vi "WPI_SolenoidSetEnum.vi"(8 "error in (no error)":errorcluster, 10 "Value":T1, 11 "SolenoidDevRef":T2={"DevStatus"={"status"=FALSE, "code"=0, "source"=""}, "Pneumatics Control Module"=0, "Forward Solenoid Channel"=enum."Invalid", "Reverse Solenoid Channel"=enum."Invalid"}) -> (0 "error out":errorcluster, 3 "SolenoidDevRef":T2={"DevStatus"={"status"=FALSE, "code"=0, "source"=""}, "Pneumatics Control Module"=0, "Forward Solenoid Channel"=enum."Invalid", "Reverse Solenoid Channel"=enum."Invalid"})   [LabVIEW 2017]
doc: "Sets the solenoid to Off, On, Forward, or Reverse. You also can wire a boolean data type to the <B>Value</B> input so that this VI specifies, when TRUE, to turn on a Single solenoid.\n\nThis software is licensed. Open the labview\\readme\\WPI Robotics Library Open Source License.txt file for more information."
uses:
  <vilib>/Rock Robotics/WPI/Solenoid/WPI_SolenoidDevRef.ctl
  <vilib>/Rock Robotics/WPI/Solenoid/WPI_SolenoidChannel.ctl
  <vilib>/Rock Robotics/WPI/Solenoid/WPI_SolenoidValue.ctl
  <vilib>/Rock Robotics/WPI/Solenoid/WPI_SolenoidCacheOp.ctl
  <vilib>/Rock Robotics/WPI/CAN/PCM/WPI_CAN_PCMGlobalOps.ctl
  <vilib>/Rock Robotics/WPI/Solenoid/WPI_SolenoidSafetyCheck.vi
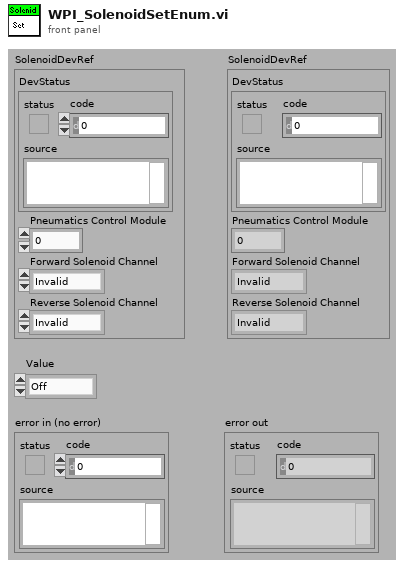
[diagram p1: front panel]
types:
  T1 = typedef "WPI_SolenoidValue.ctl" = enum16{"Off", "On", "Forward", "Reverse"}
  T2 = typedef "WPI_SolenoidDevRef.ctl" = cluster{"DevStatus":errorcluster, "Pneumatics Control Module":u8, "Forward Solenoid Channel":T3, "Reverse Solenoid Channel":T3}
  T3 = typedef "WPI_SolenoidChannel.ctl" = enum8{"Solenoid 0", "Solenoid 1", "Solenoid 2", "Solenoid 3", "Solenoid 4", "Solenoid 5", "Solenoid 6", "Solenoid 7", "Invalid"}
  T4 = typedef "WPI_SolenoidCacheOp.ctl" = enum16{"Acquire", "Release", "Status"}
  T5 = typedef "WPI_CAN_PCMGlobalOps.ctl" = enum16{"Read For Send", "Write After Receive", "Set Solenoids", "Set Closed Loop", "Clear Sticky Faults", "Get All", "Write Error", "Write After Receive Blacklist", "Set Control Frame Rate"}
  T6 = cluster{"Solenoid Status":bool[], "Battery Voltage":dbl, "Solenoid Voltage":dbl, "Compressor Current":dbl, "CompressorEnabled":bool, "StickySolenoidFault":bool, "StickyCompressorFault":bool, "SolenoidFault":bool, "CompressorFault":bool, "HardwareFault":bool, "ClosedLoopStatus":bool, "PressureStatus":bool, "Module Enabled":bool, "ClosedLoopSuggestedOutput":bool, "CAN Error":errorcluster, "Sticky Solenoid Faults":bool[]}
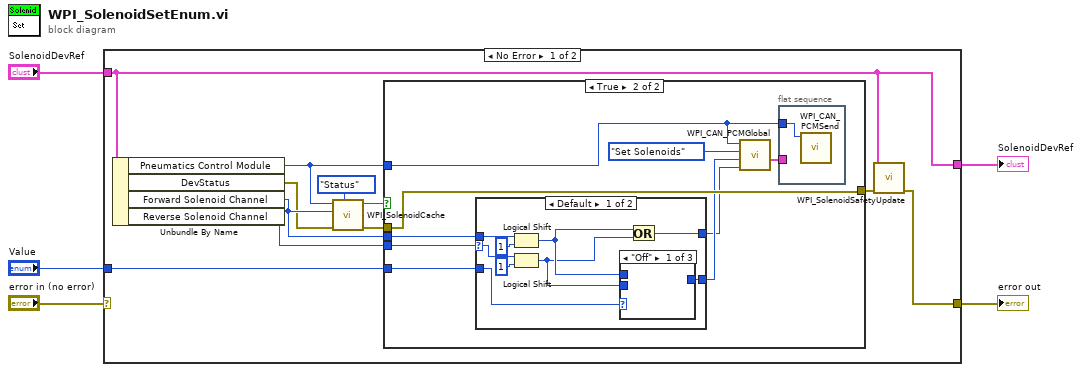
[diagram p0: block diagram]
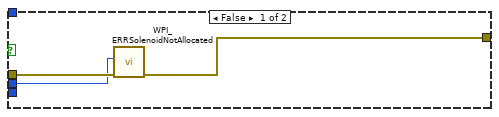
[diagram p2: hidden frame]
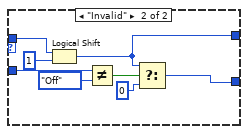
[diagram p5: hidden frame]
diagram:
  n1 = case shown="No Error" "error in (no error)" {
    selector: "error in (no error)" -> [_ w50]
    tunnel: "SolenoidDevRef" -> [w6 w49]
    tunnel: "Value" -> [w16 _]
    tunnel: [w8 w50] -> w2
    tunnel: [w6 w49] -> w1
    frame No Error {
      n2 = Unbundle By Name(w6) -> ("Pneumatics Control Module"=w15:u8, "DevStatus"=w13:errorcluster, "Forward Solenoid Channel"=w14:T3, "Reverse Solenoid Channel"=w7:T3)
      n3 = call <vilib>:"WPI_SolenoidCache.vi"("AllocatedSolenoidOp"=WPI_SolenoidCacheOp."Status", "error in (no error)"=w13, "SolenoidChannel"=w14, "Pneumatics Control Module"=w15) -> ("error out"=w11:errorcluster, "Allocated"=w12:bool)  [unwired: 6 out]
      n4 = case shown="True" w12 {
        tunnel: w16 -> [_ w28]
        tunnel: [w19 w24] -> w9
        tunnel: w15 -> [_ w21]
        tunnel: w14 -> [w17 w27]
        tunnel: w11 -> [w18 w24]
        tunnel: w7 -> [_ w26]
        frame False {
          n5 = call <vilib>:"WPI_ERRSolenoidNotAllocated.vi"("error in (no error)"=w18, "Solenoid Channel"=w17) -> ("error out"=w19:errorcluster)  [unwired: 9 in]
        }
        frame True {
          n6 = case shown="Default" w26 {
            selector: w26 -> [w35 _]
            tunnel: w28 -> [w34 w46]
            tunnel: [w33 w42] -> w23
            tunnel: w27 -> [w37 w47]
            tunnel: [w30 w43] -> w22
            frame Default {
              n7 = Logical Shift(y=w37, x=u8 1) -> (x << y=w32:u8)
              n8 = Logical Shift(y=w35, x=u8 1) -> (x << y=w31:u8)
              n9 = case shown="\"Off\"" w34 {
                tunnel: w32 -> [_ w39 _]
                tunnel: w31 -> [_ _ w40]
                tunnel: [_ w39 w40] -> w33
                frame "Off" {
                }
                frame "Forward", Default {
                }
                frame "Reverse" {
                }
              }
              n10 = Or(x=w32, y=w31) -> (x .or. y?=w30:u8)
            }
            frame "Invalid" {
              n11 = Logical Shift(y=w47, x=u8 1) -> (x << y=w43:u8)
              n12 = Not Equal?(x=w46, y=WPI_SolenoidValue."Off") -> (x != y?=w44:bool)
              n13 = Select(t=w43, s=w44, f=u8 0) -> (s? t:f=w42:u8)
            }
          }
          n14 = call <vilib>:"WPI_CAN_PCMGlobal.vi"("Solenoid Set Mask"=w22, "Solenoid Set Value"=w23, "Operation"=WPI_CAN_PCMGlobalOps."Set Solenoids", "Pneumatics Control Module (0)"=w21) -> ("Get All"=w20:T6)  [unwired: 5 in, 2 out]
          n15 = flat-sequence {
            tunnel: w21 -> [w29]
            tunnel: w20 -> [_]
            frame #0 {
              n16 = call <vilib>:"WPI_CAN_PCMSend.vi"("Pneumatics Control Module (0)"=w29) -> ()  [unwired: 10 in, 1 out]
            }
          }
        }
      }
      n17 = call <vilib>:"WPI_SolenoidSafetyUpdate.vi"("error in (no error)"=w9, "SolenoidDevRef"=w6) -> ("error out"=w8:errorcluster)  [unwired: 9 out]
    }
    frame Error {
    }
  }
  "SolenoidDevRef" <- w1
  "error out" <- w2
